vi "flag_read.vi"(8 "error in (no error)":errorcluster, 10 "flag number":i32=3) -> (0 "error out":errorcluster, 2 "flag value":bool=TRUE)   [LabVIEW 2016]
uses:
  flag_array.vi
panel:
  out "Array":bool[](array[boolean])
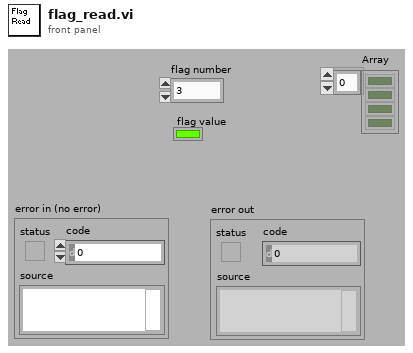
[diagram p1: front panel]
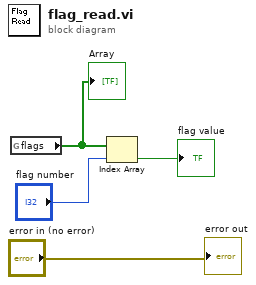
[diagram p0: block diagram]
diagram:
  n1 = global read "flag_array.vi" "flags"() -> (w1:bool[])
  "Array" <- w1
  n2 = Index Array(array=w1, index="flag number") -> (element=→"flag value":bool)
  "error out" <- "error in (no error)"
